vi "ramp from n pts.vi"(0 "start value":dbl=10.0, 7 "N intervals":i32=5, 11 "end value":dbl=20.0) -> (4 "ramp step":dbl=2.0, 8 "Values array":dbl[](array[numeric])=[10.0, 12.0, 14.0, 16.0, 18.0, 20.0], 15 "array size":i32)   [LabVIEW 2019]
doc: "This subVI creates a 1D array of values with N intervals (N+1 points) starting at \"start value\" and ending at \"end value.\"\n\nPaul K Dixon\nP3600\nCSUSB Physics"
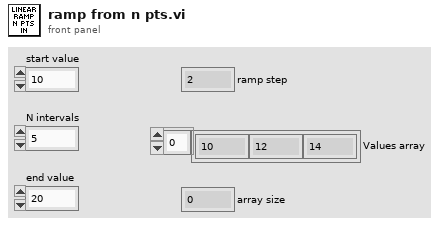
[diagram p1: front panel]
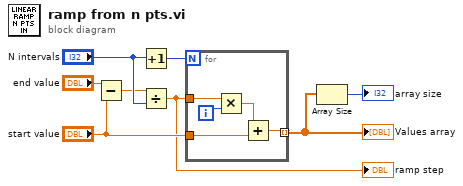
[diagram p0: block diagram]
diagram:
  n1 = Subtract(x="end value", y="start value") -> (x-y=w3:dbl)
  n2 = Increment(x="N intervals") -> (x+1=w4:i32)
  n3 = Divide(x=w3, y="N intervals") -> (x/y=w6:dbl)
  "ramp step" <- w6
  n4 = for {
    N: w4 -> [_]
    tunnel: w6 -> [w12]
    tunnel: [w10] -> w2 mode=indexing
    tunnel: "start value" -> [w9]
    i -> [w13]
    n5 = Multiply(x=w12, y=w13) -> (x*y=w11:dbl)
    n6 = Add(x=w11, y=w9) -> (x+y=w10:dbl)
  }
  "Values array" <- w2
  n7 = Array Size(array=w2) -> (size(s)=→"array size":i32)
